vi "Persistence parser.vi"(10 "Incoming Data in":u8[](array[numeric])) -> (0 "AIHTH":u8, 1 "AIHTL":u8, 2 "AILTH":u8, 3 "AILTL":u8, 4 "PERS":u8)   [LabVIEW 2014, in "AMS TS3472 Light Sensor.lvlib" / "AMS TCS3472.lvclass"]
uses:
  AMS TCS3472.lvclass
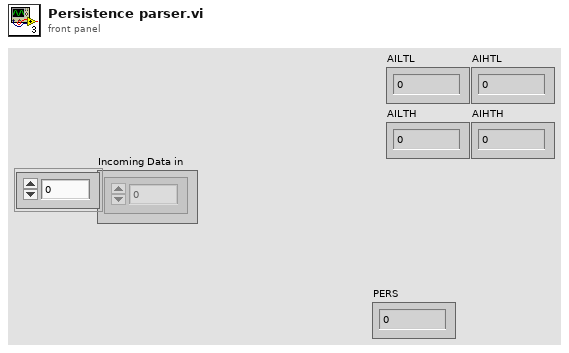
[diagram p1: front panel]
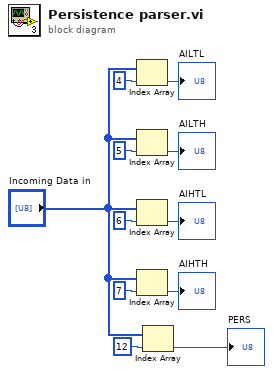
[diagram p0: block diagram]
diagram:
  n1 = Index Array(array="Incoming Data in", index=4) -> (element=→"AILTL":u8)
  n2 = Index Array(array="Incoming Data in", index=5) -> (element=→"AILTH":u8)
  n3 = Index Array(array="Incoming Data in", index=6) -> (element=→"AIHTL":u8)
  n4 = Index Array(array="Incoming Data in", index=7) -> (element=→"AIHTH":u8)
  n5 = Index Array(array="Incoming Data in", index=12) -> (element=→"PERS":u8)
